vi "Load Image From File (Path).vi"(8 "error in (no error)":errorcluster, 11 "Path In":path) -> (0 "error out":errorcluster, 2 "Image":T1, 3 "Path Out":path)   [LabVIEW 2020, in "G-Image.lvlib"]
doc: "Load an image file from disk, and return it as a LabVIEW picture."
uses:
  G-Image.lvlib
  <vilib>/picture/picture.llb/imagedata.ctl
  Private/Result To Error.vi
  Private/Copy Image To Pixmap.vi
  Private/RGBA To ARGB.vi
  <vilib>/Utility/error.llb/Error Cluster From Error Code.vi
  <vilib>/picture/picture.llb/Create Mask By Alpha.vi
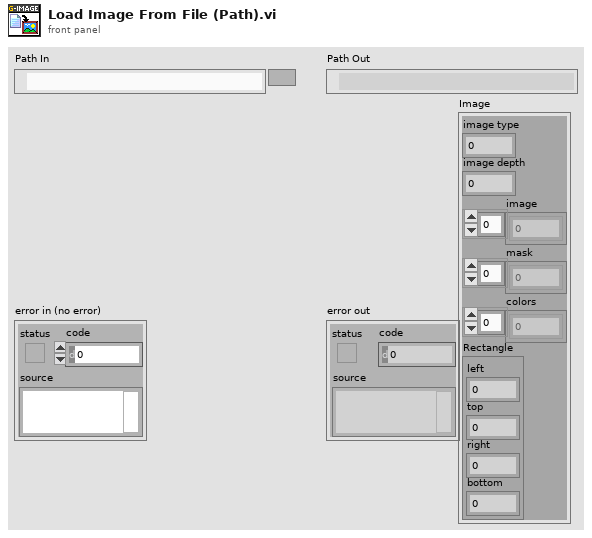
[diagram p1: front panel]
types:
  T1 = typedef "imagedata.ctl" = cluster{"image type":i32, "image depth":i32, "image":u8[], "mask":u8[], "colors":u32[], "Rectangle":cluster{"left":i16, "top":i16, "right":i16, "bottom":i16}}
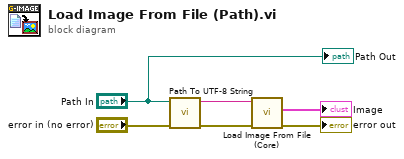
[diagram p0: block diagram]
diagram:
  n1 = call "Path To UTF-8 String.vi"("error in"="error in (no error)", "Path"="Path In") -> ("error out"=w2:errorcluster, "UTF-8 String"=w5:string)  [unwired: 8 in]
  n2 = call "Load Image From File (Core).vi"("error in (no error)"=w2, "Path In"=w5) -> ("error out"=→"error out":errorcluster, "Image"=→"Image":T1)  [unwired: 7 in, 1 out]
  "Path Out" <- "Path In"
